vi "Read Target-FIFO Single channel.vi"(1 "FIFO In":refnum<k21>="FIFO-000", 9 "ready for input":bool) -> (4 "16xIQData":T1(array[cluster]) {"I" format="%.18g"; "Q" format="%.18g"}, 10 "Output Valid":bool)   [LabVIEW 2015, in "DDC_7976R_v1.lvlib"]
uses:
  DDC_7976R_v1.lvlib
types:
  T1 = cluster{"I":fxp<+/-,18,1>, "Q":fxp<+/-,18,1>, "overflow":bool}[]
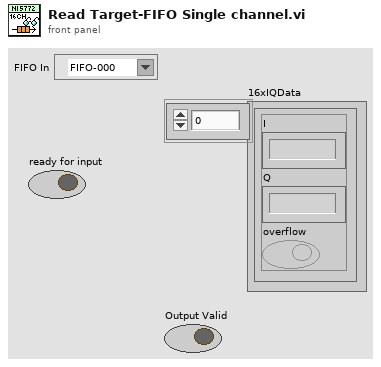
[diagram p1: front panel]
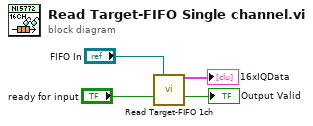
[diagram p0: block diagram]
diagram:
  n1 = call "Read Target-FIFO 1ch.vi"("FIFO In"="FIFO In", "ready for input"="ready for input") -> ("16xIQData"=→"16xIQData":T1, "Output Valid"=→"Output Valid":bool)  [unwired: 12 in]
